vi "SlaveFrame.vi"(0 "buf":u8[](array[numeric]) format="%02x", 5 "数组大小":i32, 7 "Mode":bool) -> (1 "数据帧分析":string, 2 "接收显示":string, 3 "校验成功":bool, 4 "从机编号":u8 format="%02x", 6 "功能码":u8 format="%02x", 8 "起始地址":u16 format="%04x", 10 "寄存器/线圈数量":u16 format="%04x", 14 "数据值索引":u16 format="%04x", 15 "输入数量/字节数":u16 format="%04x")   [LabVIEW 2015]
doc: "Mode = 1? RTU；ASCII;"
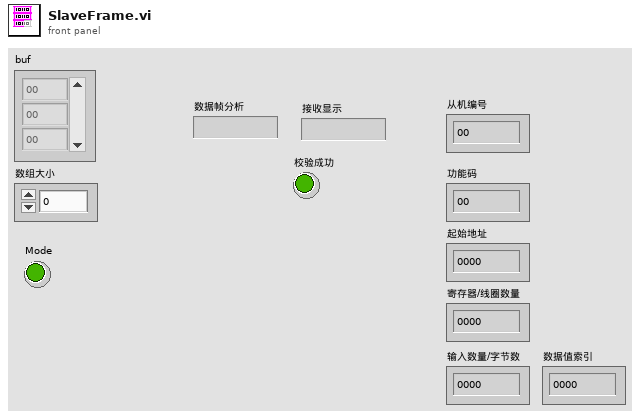
[diagram p1: front panel]
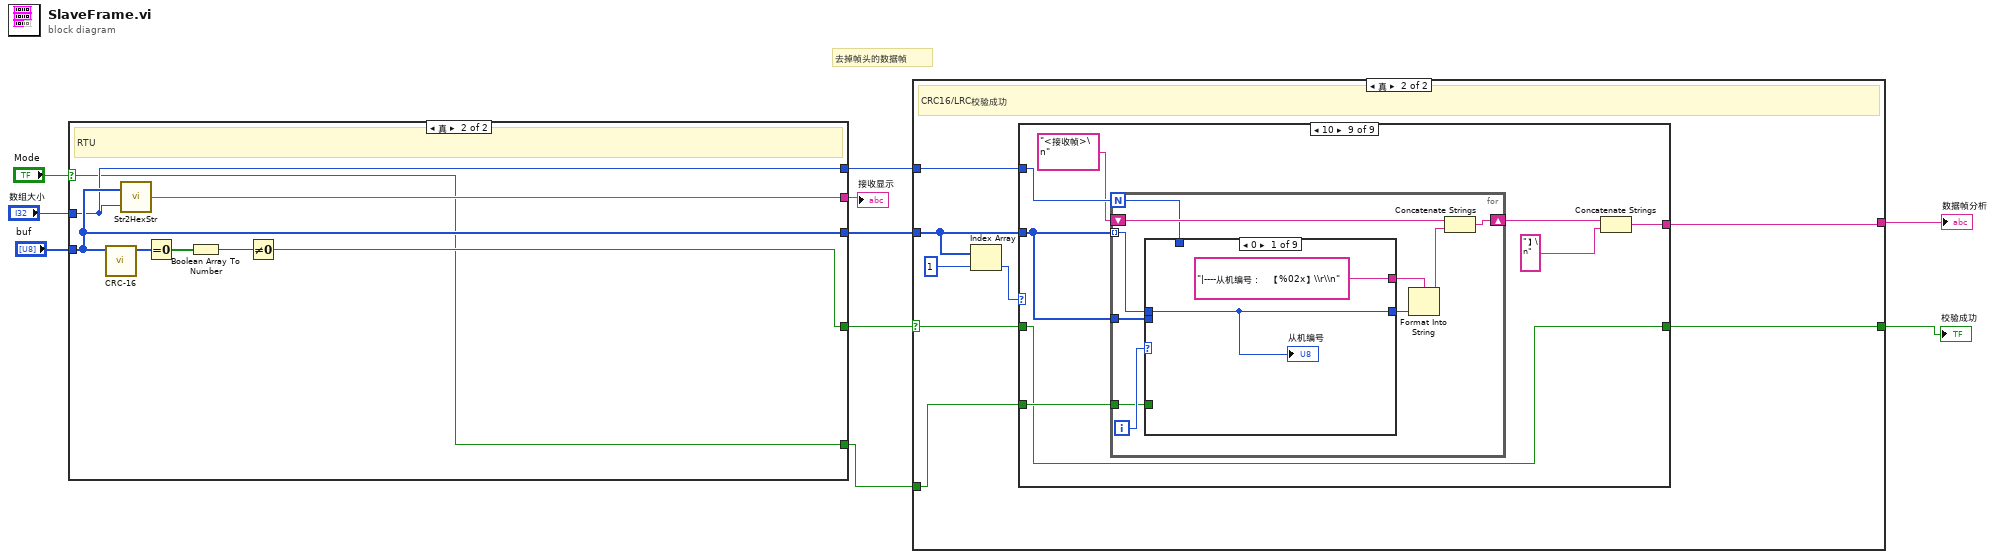
[diagram p0: block diagram]
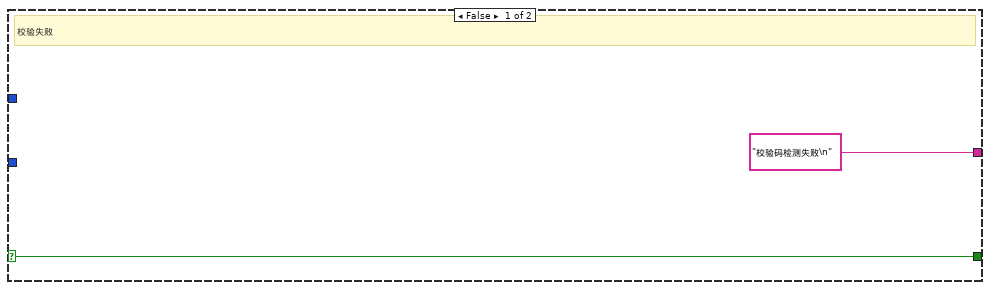
[diagram p2: hidden frame]
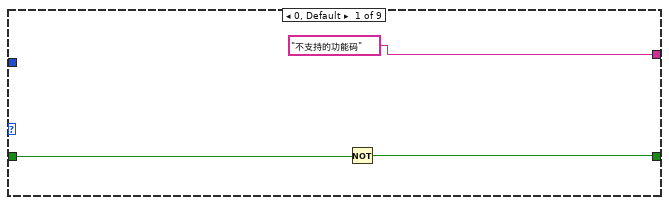
[diagram p3: hidden frame]
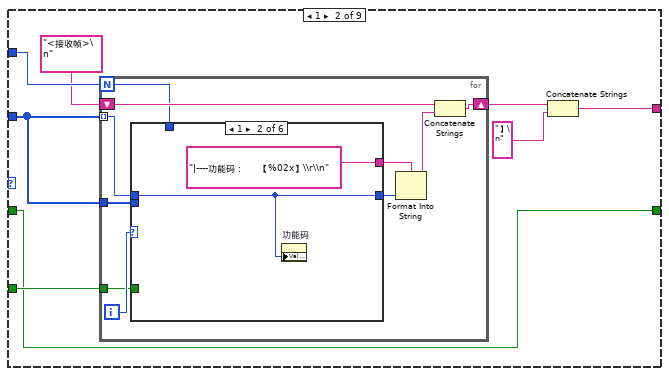
[diagram p4: hidden frame]
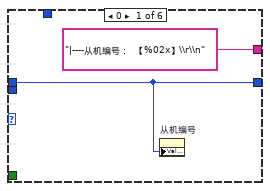
[diagram p5: hidden frame]
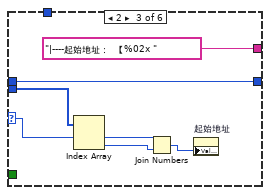
[diagram p6: hidden frame]
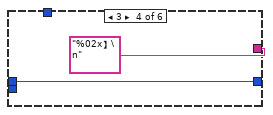
[diagram p7: hidden frame]
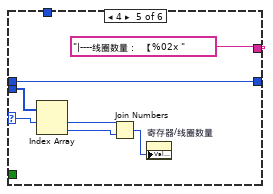
[diagram p8: hidden frame]
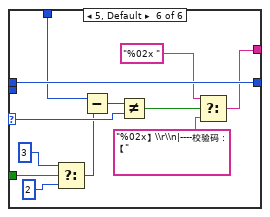
[diagram p9: hidden frame]
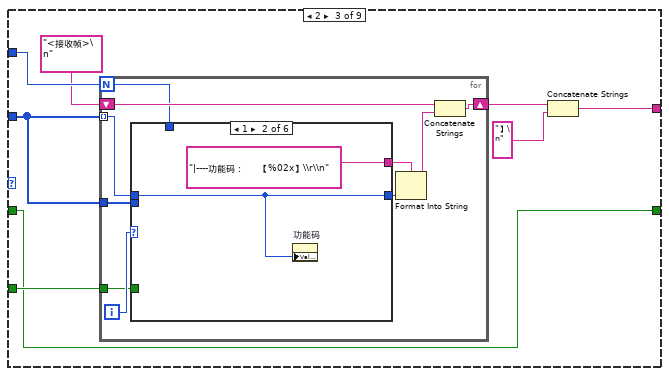
[diagram p10: hidden frame]
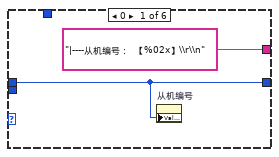
[diagram p11: hidden frame]
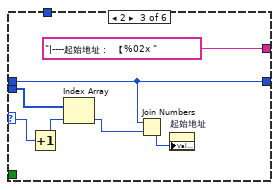
[diagram p12: hidden frame]
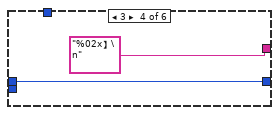
[diagram p13: hidden frame]
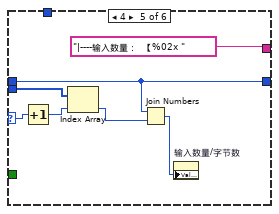
[diagram p14: hidden frame]
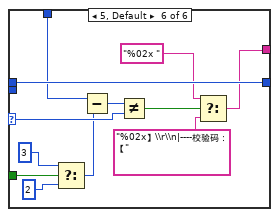
[diagram p15: hidden frame]
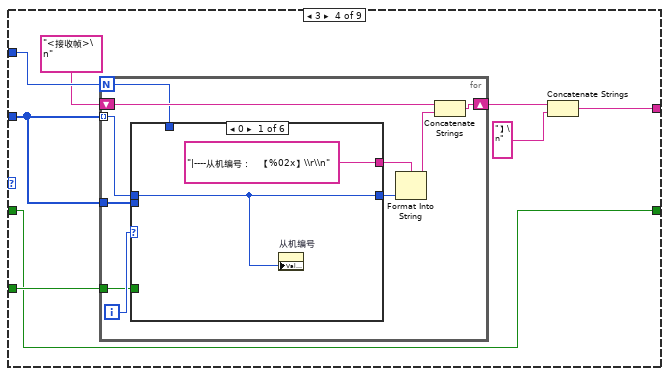
[diagram p16: hidden frame]
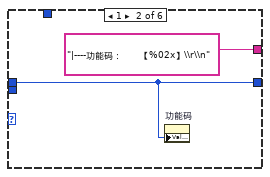
[diagram p17: hidden frame]
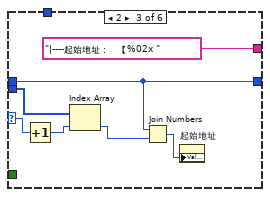
[diagram p18: hidden frame]
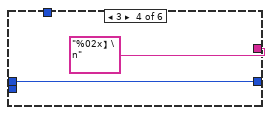
[diagram p19: hidden frame]
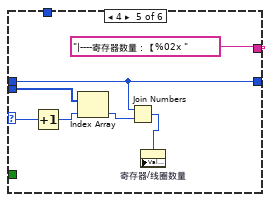
[diagram p20: hidden frame]
diagram:
  # "去掉帧头的数据帧"
  n1 = case shown="真" "Mode" {
    selector: "Mode" -> [w11 w46]
    tunnel: "buf" -> [w24 w48]
    tunnel: "数组大小" -> [_ w47]
    tunnel: [w15 w50] -> w9
    tunnel: [w14 w49] -> w2
    tunnel: [w13 w48] -> w8
    tunnel: [w12 w47] -> w6
    tunnel: [w11 w46] -> w3
    frame False {
      # "ASCII模式"
      n2 = Byte Array To String(unsigned byte array=w24) -> (string=w23:string)
      n3 = Match Pattern(string=w23, regular expression="[:]+[^]+[\\r\\n]") -> (match substring=w15:string)  [unwired: 1 in, 3 out]
      n4 = Match Pattern(string=w23, regular expression="[~:]+[^]+[~\\r\\n]") -> (match substring=w18:string)  [unwired: 1 in, 3 out]
      n5 = String To Byte Array(string=w18) -> (unsigned byte array=w21:u8[])
      n6 = Decimate 1D Array(w21) -> (w20:u8[], w19:u8[])
      n7 = for {
        tunnel: w20 -> [w32] mode=indexing
        tunnel: w19 -> [w30] mode=indexing
        tunnel: [w25] -> w13 mode=indexing
        w29 = u8 57
        w28 = u8 48
        n8 = In Range and Coerce(upper limit=w29, x=w32, lower limit=w28) -> (In Range?=w33:bool)  [unwired: 1 out]
        n9 = In Range and Coerce(upper limit=w29, x=w30, lower limit=w28) -> (In Range?=w31:bool)  [unwired: 1 out]
        n10 = case shown="假" w33 {
          tunnel: w32 -> [w41 w45]
          tunnel: w28 -> [_ w44]
          tunnel: [w40 w43] -> w27
          frame False {
            n11 = Subtract(x=w41, y=u8 55) -> (x-y=w40:u8)
          }
          frame True {
            n12 = Subtract(x=w45, y=w44) -> (x-y=w43:u8)
          }
        }
        n13 = case shown="假" w31 {
          tunnel: w30 -> [w35 w39]
          tunnel: [w34 w38] -> w26
          tunnel: w28 -> [_ w37]
          frame False {
            n14 = Subtract(x=w35, y=u8 55) -> (x-y=w34:u8)
          }
          frame True {
            n15 = Subtract(x=w39, y=w37) -> (x-y=w38:u8)
          }
        }
        n16 = formula code="uInt8 result;\nHi<<=4;\nresult=Hi|Lo;"("Hi"=w27, "Lo"=w26) -> ("result"=w25:u8)
      }
      n17 = Array Size(array=w13) -> (size(s)=w12:i32)
      n18 = call "LRC-8.vi"("Frame in"=w13) -> ("LRC-8"=w16:u8)  [unwired: 2 in]
      n19 = Equal To 0?(x=w16) -> (x = 0?=w14:bool)
    }
    frame True {
      # "RTU"
      n20 = call "CRC-16.vi"("Frame in"=w48) -> ("CRC-16"=w53:u8[])  [unwired: 6 in]
      n21 = call "Str2HexStr.vi"("数组大小"=w47, "数组"=w48) -> ("OutStr"=w50:string)
      n22 = Equal To 0?(x=w53) -> (x = 0?=w52:bool[])
      n23 = Boolean Array To Number(Boolean array=w52) -> (number=w51:u32)
      n24 = Not Equal To 0?(x=w51) -> (x != 0?=w49:bool)
    }
  }
  "接收显示" <- w9
  n25 = case shown="真" w2 {
    selector: w2 -> [w54 w56]
    tunnel: w8 -> [_ w60]
    tunnel: ["校验码检测失败\n" w63] -> w5
    tunnel: w6 -> [_ w62]
    tunnel: w3 -> [_ w61]
    tunnel: [w54 w57] -> w1
    frame False {
      # "校验失败"
    }
    frame True {
      # "CRC16/LRC校验成功"
      n26 = Index Array(array=w60, index=1) -> (element=w58:u8)
      n27 = case shown="10" w58 {
        tunnel: ["不支持的功能码" w74 w124 w174 w224 w274 w320 w366 w430] -> w63
        tunnel: w62 -> [_ w73 w123 w173 w223 w273 w319 w365 w429]
        tunnel: w61 -> [_ w72 w122 w172 w222 w272 w318 w364 w428]
        tunnel: w60 -> [_ w71 w121 w171 w221 w271 w317 w363 w427]
        tunnel: [w64 w67 w117 w167 w217 w267 w313 w359 w423] -> w57
        tunnel: w56 -> [w65 w67 w117 w167 w217 w267 w313 w359 w423]
        frame 0, Default {
          n28 = Not(x=w65) -> (.not. x?=w64:bool)
        }
        frame 1 {
          n29 = for {
            N: w73 -> [w76]
            shift-right: [w84] -> w69
            shift-left: "<接收帧>\n" -> [w83]
            tunnel: w71 -> [w77] mode=indexing
            tunnel: w71 -> [w79]
            tunnel: w72 -> [w75]
            i -> [w80]
            n30 = case shown="1" w80 {
              selector: w80 -> [_ _ w93 _ w100 w109]
              tunnel: ["|----从机编号：  【%02x】\\r\\n" "|----功能码：     【%02x】\\r\\n" "|----起始地址：  【%02x " "%02x】\n" "|----线圈数量：  【%02x " w111] -> w82
              tunnel: w79 -> [_ _ w92 _ w99 _]
              tunnel: [w85 w87 w95 w96 w103 w116] -> w78
              tunnel: w77 -> [w85 w87 w95 w96 w103 w116]
              tunnel: w76 -> [_ _ _ _ _ w115]
              tunnel: w75 -> [_ _ _ _ _ w108]
              frame 0 {
                n31 = property on="从机编号" class="DigNum (严格)"("Value"=w85) -> ()  [unwired: 2 in, 2 out]
              }
              frame 1 {
                n32 = property on="功能码" class="DigNum (严格)"("Value"=w87) -> ()  [unwired: 2 in, 2 out]
              }
              frame 2 {
                n33 = Index Array(array=w92, index #1=w93) -> (element #1=w91:u8, element #2=w90:u8)  [unwired: 1 in]
                n34 = Join Numbers(hi=w91, lo=w90) -> ((hi.lo)=w89:u16)
                n35 = property on="起始地址" class="DigNum (严格)"("Value"=w89) -> ()  [unwired: 2 in, 2 out]
              }
              frame 3 {
              }
              frame 4 {
                n36 = Index Array(array=w99, index #1=w100) -> (element #1=w102:u8, element #2=w101:u8)  [unwired: 1 in]
                n37 = Join Numbers(hi=w102, lo=w101) -> ((hi.lo)=w98:u16)
                n38 = property on="寄存器/线圈数量" class="DigNum (严格)"("Value"=w98) -> ()  [unwired: 2 in, 2 out]
              }
              frame 5, Default {
                n39 = Select(t=3, s=w108, f=2) -> (s? t:f=w106:i32)
                n40 = Subtract(x=w115, y=w106) -> (x-y=w114:i32)
                n41 = Not Equal?(x=w114, y=w109) -> (x != y?=w113:bool)
                n42 = Select(t="%02x ", s=w113, f="%02x】\\r\\n|----校验码：     【") -> (s? t:f=w111:string)
              }
            }
            n43 = Format Into String(format string=w82, w78) -> (resulting string=w81:string)  [unwired: 2 in, 1 out]
            n44 = Concatenate Strings(w83, w81) -> (w84:string)
          }
          n45 = Concatenate Strings(w69, "】\n") -> (w74:string)
        }
        frame 2 {
          n46 = for {
            N: w123 -> [w126]
            shift-right: [w134] -> w119
            shift-left: "<接收帧>\n" -> [w133]
            tunnel: w121 -> [w127] mode=indexing
            tunnel: w121 -> [w129]
            tunnel: w122 -> [w125]
            i -> [w130]
            n47 = case shown="1" w130 {
              selector: w130 -> [_ _ w142 _ w151 w159]
              tunnel: ["|----从机编号：  【%02x】\\r\\n" "|----功能码：     【%02x】\\r\\n" "|----起始地址：  【%02x " "%02x】\n" "|----输入数量：  【%02x " w161] -> w132
              tunnel: w129 -> [_ _ w144 _ w150 _]
              tunnel: [w135 w137 w139 w146 w149 w166] -> w128
              tunnel: w127 -> [w135 w137 w139 w146 w149 w166]
              tunnel: w126 -> [_ _ _ _ _ w165]
              tunnel: w125 -> [_ _ _ _ _ w158]
              frame 0 {
                n48 = property on="从机编号" class="DigNum (严格)"("Value"=w135) -> ()  [unwired: 2 in, 2 out]
              }
              frame 1 {
                n49 = property on="功能码" class="DigNum (严格)"("Value"=w137) -> ()  [unwired: 2 in, 2 out]
              }
              frame 2 {
                n50 = Increment(x=w142) -> (x+1=w141:i32)
                n51 = Index Array(array=w144, index=w141) -> (element=w140:u8)
                n52 = Join Numbers(hi=w139, lo=w140) -> ((hi.lo)=w143:u16)
                n53 = property on="起始地址" class="DigNum (严格)"("Value"=w143) -> ()  [unwired: 2 in, 2 out]
              }
              frame 3 {
              }
              frame 4 {
                n54 = Increment(x=w151) -> (x+1=w153:i32)
                n55 = Index Array(array=w150, index=w153) -> (element=w152:u8)
                n56 = Join Numbers(hi=w149, lo=w152) -> ((hi.lo)=w148:u16)
                n57 = property on="输入数量/字节数" class="DigNum (严格)"("Value"=w148) -> ()  [unwired: 2 in, 2 out]
              }
              frame 5, Default {
                n58 = Select(t=3, s=w158, f=2) -> (s? t:f=w156:i32)
                n59 = Subtract(x=w165, y=w156) -> (x-y=w164:i32)
                n60 = Not Equal?(x=w164, y=w159) -> (x != y?=w163:bool)
                n61 = Select(t="%02x ", s=w163, f="%02x】\\r\\n|----校验码：     【") -> (s? t:f=w161:string)
              }
            }
            n62 = Format Into String(format string=w132, w128) -> (resulting string=w131:string)  [unwired: 2 in, 1 out]
            n63 = Concatenate Strings(w133, w131) -> (w134:string)
          }
          n64 = Concatenate Strings(w119, "】\n") -> (w124:string)
        }
        frame 3 {
          n65 = for {
            N: w173 -> [w176]
            shift-right: [w184] -> w169
            shift-left: "<接收帧>\n" -> [w183]
            tunnel: w171 -> [w177] mode=indexing
            tunnel: w171 -> [w179]
            tunnel: w172 -> [w175]
            i -> [w180]
            n66 = case shown="0" w180 {
              selector: w180 -> [_ _ w192 _ w199 w209]
              tunnel: ["|----从机编号：   【%02x】\\r\\n" "|----功能码：      【%02x】\\r\\n" "|----起始地址：   【%02x " "%02x】\n" "|----寄存器数量：【%02x " w211] -> w182
              tunnel: w179 -> [_ _ w191 _ w200 _]
              tunnel: [w185 w187 w190 w196 w201 w216] -> w178
              tunnel: w177 -> [w185 w187 w190 w196 w201 w216]
              tunnel: w176 -> [_ _ _ _ _ w215]
              tunnel: w175 -> [_ _ _ _ _ w208]
              frame 0 {
                n67 = property on="从机编号" class="DigNum (严格)"("Value"=w185) -> ()  [unwired: 2 in, 2 out]
              }
              frame 1 {
                n68 = property on="功能码" class="DigNum (严格)"("Value"=w187) -> ()  [unwired: 2 in, 2 out]
              }
              frame 2 {
                n69 = Increment(x=w192) -> (x+1=w194:i32)
                n70 = Index Array(array=w191, index=w194) -> (element=w193:u8)
                n71 = Join Numbers(hi=w190, lo=w193) -> ((hi.lo)=w189:u16)
                n72 = property on="起始地址" class="DigNum (严格)"("Value"=w189) -> ()  [unwired: 2 in, 2 out]
              }
              frame 3 {
              }
              frame 4 {
                n73 = Increment(x=w199) -> (x+1=w203:i32)
                n74 = Index Array(array=w200, index=w203) -> (element=w202:u8)
                n75 = Join Numbers(hi=w201, lo=w202) -> ((hi.lo)=w198:u16)
                n76 = property on="寄存器/线圈数量" class="DigNum (严格)"("Value"=w198) -> ()  [unwired: 2 in, 2 out]
              }
              frame 5, Default {
                n77 = Select(t=3, s=w208, f=2) -> (s? t:f=w206:i32)
                n78 = Subtract(x=w215, y=w206) -> (x-y=w214:i32)
                n79 = Not Equal?(x=w214, y=w209) -> (x != y?=w213:bool)
                n80 = Select(t="%02x ", s=w213, f="%02x】\\r\\n|----校验码：      【") -> (s? t:f=w211:string)
              }
            }
            n81 = Format Into String(format string=w182, w178) -> (resulting string=w181:string)  [unwired: 2 in, 1 out]
            n82 = Concatenate Strings(w183, w181) -> (w184:string)
          }
          n83 = Concatenate Strings(w169, "】\n") -> (w174:string)
        }
        frame 4 {
          n84 = for {
            N: w223 -> [w226]
            shift-right: [w234] -> w219
            shift-left: "<接收帧>\n" -> [w233]
            tunnel: w221 -> [w227] mode=indexing
            tunnel: w221 -> [w229]
            tunnel: w222 -> [w225]
            i -> [w230]
            n85 = case shown="5, 默认" w230 {
              selector: w230 -> [_ _ w241 _ w248 w259]
              tunnel: ["|----从机编号：   【%02x】\\r\\n" "|----功能码：      【%02x】\\r\\n" "|----起始地址：   【%02x " "%02x】\n" "|----寄存器数量：【%02x " w261] -> w232
              tunnel: w229 -> [_ _ w240 _ w249 _]
              tunnel: [w235 w237 w239 w246 w250 w266] -> w228
              tunnel: w227 -> [w235 w237 w239 w246 w250 w266]
              tunnel: w226 -> [_ _ _ _ _ w265]
              tunnel: w225 -> [_ _ _ _ _ w258]
              frame 0 {
                n86 = property on="从机编号" class="DigNum (严格)"("Value"=w235) -> ()  [unwired: 2 in, 2 out]
              }
              frame 1 {
                n87 = property on="功能码" class="DigNum (严格)"("Value"=w237) -> ()  [unwired: 2 in, 2 out]
              }
              frame 2 {
                n88 = Increment(x=w241) -> (x+1=w243:i32)
                n89 = Index Array(array=w240, index=w243) -> (element=w242:u8)
                n90 = Join Numbers(hi=w239, lo=w242) -> ((hi.lo)=w244:u16)
                n91 = property on="起始地址" class="DigNum (严格)"("Value"=w244) -> ()  [unwired: 2 in, 2 out]
              }
              frame 3 {
              }
              frame 4 {
                n92 = Increment(x=w248) -> (x+1=w253:i32)
                n93 = Index Array(array=w249, index=w253) -> (element=w252:u8)
                n94 = Join Numbers(hi=w250, lo=w252) -> ((hi.lo)=w251:u16)
                n95 = property on="寄存器/线圈数量" class="DigNum (严格)"("Value"=w251) -> ()  [unwired: 2 in, 2 out]
              }
              frame 5, Default {
                n96 = Select(t=3, s=w258, f=2) -> (s? t:f=w256:i32)
                n97 = Subtract(x=w265, y=w256) -> (x-y=w264:i32)
                n98 = Not Equal?(x=w264, y=w259) -> (x != y?=w263:bool)
                n99 = Select(t="%02x ", s=w263, f="%02x】\\r\\n|----校验码：      【") -> (s? t:f=w261:string)
              }
            }
            n100 = Format Into String(format string=w232, w228) -> (resulting string=w231:string)  [unwired: 2 in, 1 out]
            n101 = Concatenate Strings(w233, w231) -> (w234:string)
          }
          n102 = Concatenate Strings(w219, "】\n") -> (w224:string)
        }
        frame 5 {
          n103 = for {
            N: w273 -> [w276]
            shift-right: [w284] -> w269
            shift-left: "<接收帧>\n" -> [w283]
            tunnel: w271 -> [w277] mode=indexing
            tunnel: w271 -> [w279]
            tunnel: w272 -> [w275]
            i -> [w280]
            n104 = case shown="0" w280 {
              selector: w280 -> [_ _ w291 _ w298 w305]
              tunnel: ["|----从机编号：   【%02x】\\r\\n" "|----功能码：      【%02x】\\r\\n" "|----起始地址：   【%02x " "%02x】\n" "|----数据值：      【%02x " w307] -> w282
              tunnel: w279 -> [_ _ w290 _ _ _]
              tunnel: [w285 w287 w289 w296 w299 w312] -> w278
              tunnel: w277 -> [w285 w287 w289 w296 w299 w312]
              tunnel: w276 -> [_ _ _ _ _ w311]
              tunnel: w275 -> [_ _ _ _ _ w304]
              frame 0 {
                n105 = property on="从机编号" class="DigNum (严格)"("Value"=w285) -> ()  [unwired: 2 in, 2 out]
              }
              frame 1 {
                n106 = property on="功能码" class="DigNum (严格)"("Value"=w287) -> ()  [unwired: 2 in, 2 out]
              }
              frame 2 {
                n107 = Increment(x=w291) -> (x+1=w293:i32)
                n108 = Index Array(array=w290, index=w293) -> (element=w292:u8)
                n109 = Join Numbers(hi=w289, lo=w292) -> ((hi.lo)=w294:u16)
                n110 = property on="起始地址" class="DigNum (严格)"("Value"=w294) -> ()  [unwired: 2 in, 2 out]
              }
              frame 3 {
              }
              frame 4 {
                n111 = property on="数据值索引" class="DigNum (严格)"("Value"=w298) -> ()  [unwired: 2 in, 2 out]
              }
              frame 5, Default {
                n112 = Select(t=3, s=w304, f=2) -> (s? t:f=w302:i32)
                n113 = Subtract(x=w311, y=w302) -> (x-y=w310:i32)
                n114 = Not Equal?(x=w310, y=w305) -> (x != y?=w309:bool)
                n115 = Select(t="%02x ", s=w309, f="%02x】\\r\\n|----校验码：      【") -> (s? t:f=w307:string)
              }
            }
            n116 = Format Into String(format string=w282, w278) -> (resulting string=w281:string)  [unwired: 2 in, 1 out]
            n117 = Concatenate Strings(w283, w281) -> (w284:string)
          }
          n118 = Concatenate Strings(w269, "】\n") -> (w274:string)
        }
        frame 6 {
          n119 = for {
            N: w319 -> [w322]
            shift-right: [w330] -> w315
            shift-left: "<接收帧>\n" -> [w329]
            tunnel: w317 -> [w323] mode=indexing
            tunnel: w317 -> [w325]
            tunnel: w318 -> [w321]
            i -> [w326]
            n120 = case shown="0" w326 {
              selector: w326 -> [_ _ w337 _ w344 w351]
              tunnel: ["|----从机编号：   【%02x】\\r\\n" "|----功能码：      【%02x】\\r\\n" "|----寄存器地址：【%02x " "%02x】\n" "|----寄存器值：   【%02x " w353] -> w328
              tunnel: w325 -> [_ _ w336 _ _ _]
              tunnel: [w331 w333 w335 w342 w345 w358] -> w324
              tunnel: w323 -> [w331 w333 w335 w342 w345 w358]
              tunnel: w322 -> [_ _ _ _ _ w357]
              tunnel: w321 -> [_ _ _ _ _ w350]
              frame 0 {
                n121 = property on="从机编号" class="DigNum (严格)"("Value"=w331) -> ()  [unwired: 2 in, 2 out]
              }
              frame 1 {
                n122 = property on="功能码" class="DigNum (严格)"("Value"=w333) -> ()  [unwired: 2 in, 2 out]
              }
              frame 2 {
                n123 = Increment(x=w337) -> (x+1=w339:i32)
                n124 = Index Array(array=w336, index=w339) -> (element=w338:u8)
                n125 = Join Numbers(hi=w335, lo=w338) -> ((hi.lo)=w340:u16)
                n126 = property on="起始地址" class="DigNum (严格)"("Value"=w340) -> ()  [unwired: 2 in, 2 out]
              }
              frame 3 {
              }
              frame 4 {
                n127 = property on="数据值索引" class="DigNum (严格)"("Value"=w344) -> ()  [unwired: 2 in, 2 out]
              }
              frame 5, Default {
                n128 = Select(t=3, s=w350, f=2) -> (s? t:f=w348:i32)
                n129 = Subtract(x=w357, y=w348) -> (x-y=w356:i32)
                n130 = Not Equal?(x=w356, y=w351) -> (x != y?=w355:bool)
                n131 = Select(t="%02x ", s=w355, f="%02x】\\r\\n|----校验码：      【") -> (s? t:f=w353:string)
              }
            }
            n132 = Format Into String(format string=w328, w324) -> (resulting string=w327:string)  [unwired: 2 in, 1 out]
            n133 = Concatenate Strings(w329, w327) -> (w330:string)
          }
          n134 = Concatenate Strings(w315, "】\n") -> (w320:string)
        }
        frame 15 {
          n135 = for {
            N: w365 -> [w368]
            shift-right: [w376] -> w361
            shift-left: "<接收帧>\n" -> [w375]
            tunnel: w363 -> [w369] mode=indexing
            tunnel: w363 -> [w371]
            tunnel: w364 -> [w367]
            i -> [w372]
            n136 = case shown="8, 默认" w372 {
              selector: w372 -> [_ _ w383 _ w393 _ _ w401 w415]
              tunnel: ["|----从机编号：   【%02x】\\r\\n" "|----功能码：      【%02x】\\r\\n" "|----起始地址：   【%02x " "%02x】\n" "|----输出数量：   【%02x " "%02x】\n" "|----字节数：      【%02x】 \\r\\n" w403 w417] -> w374
              tunnel: w371 -> [_ _ w382 _ w392 _ _ w408 _]
              tunnel: [w377 w379 w381 w388 w391 w397 w399 w410 w422] -> w370
              tunnel: w369 -> [w377 w379 w381 w388 w391 w397 w399 w410 w422]
              tunnel: w368 -> [_ _ _ _ _ _ _ _ w421]
              tunnel: w367 -> [_ _ _ _ _ _ _ _ w414]
              frame 0 {
                n137 = property on="从机编号" class="DigNum (严格)"("Value"=w377) -> ()  [unwired: 2 in, 2 out]
              }
              frame 1 {
                n138 = property on="功能码" class="DigNum (严格)"("Value"=w379) -> ()  [unwired: 2 in, 2 out]
              }
              frame 2 {
                n139 = Increment(x=w383) -> (x+1=w385:i32)
                n140 = Index Array(array=w382, index=w385) -> (element=w384:u8)
                n141 = Join Numbers(hi=w381, lo=w384) -> ((hi.lo)=w386:u16)
                n142 = property on="起始地址" class="DigNum (严格)"("Value"=w386) -> ()  [unwired: 2 in, 2 out]
              }
              frame 3 {
              }
              frame 4 {
                n143 = Increment(x=w393) -> (x+1=w395:i32)
                n144 = Index Array(array=w392, index=w395) -> (element=w394:u8)
                n145 = Join Numbers(hi=w391, lo=w394) -> ((hi.lo)=w390:u16)
                n146 = property on="寄存器/线圈数量" class="DigNum (严格)"("Value"=w390) -> ()  [unwired: 2 in, 2 out]
              }
              frame 5 {
              }
              frame 6 {
                n147 = property on="输入数量/字节数" class="DigNum (严格)"("Value"=w399) -> ()  [unwired: 2 in, 2 out]
              }
              frame 7 {
                n148 = Decrement(x=w401) -> (x-1=w409:i32)
                n149 = Index Array(array=w408, index=w409) -> (element=w407:u8)
                n150 = Greater?(x=w407, y=1) -> (0:w405:bool)
                n151 = Select(t="|----数据值：      【%02x ", s=w405, f="|----数据值：      【%02x】\n|----校验码：      【") -> (s? t:f=w403:string)
                n152 = property on="数据值索引" class="DigNum (严格)"("Value"=w401) -> ()  [unwired: 2 in, 2 out]
              }
              frame 8, Default {
                n153 = Select(t=3, s=w414, f=2) -> (s? t:f=w412:i32)
                n154 = Subtract(x=w421, y=w412) -> (x-y=w420:i32)
                n155 = Not Equal?(x=w420, y=w415) -> (x != y?=w419:bool)
                n156 = Select(t="%02x ", s=w419, f="%02x】\\r\\n|----校验码：      【") -> (s? t:f=w417:string)
              }
            }
            n157 = Format Into String(format string=w374, w370) -> (resulting string=w373:string)  [unwired: 2 in, 1 out]
            n158 = Concatenate Strings(w375, w373) -> (w376:string)
          }
          n159 = Concatenate Strings(w361, "】\n") -> (w366:string)
        }
        frame 16 {
          n160 = for {
            N: w429 -> [w432]
            shift-right: [w440] -> w425
            shift-left: "<接收帧>\n" -> [w439]
            tunnel: w427 -> [w433] mode=indexing
            tunnel: w427 -> [w435]
            tunnel: w428 -> [w431]
            i -> [w436]
            n161 = case shown="0" w436 {
              selector: w436 -> [_ _ w448 _ w457 _ _ w465 w472]
              tunnel: ["|----从机编号：   【%02x】\\r\\n" "|----功能码：      【%02x】\\r\\n" "|----起始地址：   【%02x " "%02x】\n" "|----寄存器数量：【%02x " "%02x】\n" "|----字节数：      【%02x】 \\r\\n" "|----数据值：      【%02x " w474] -> w438
              tunnel: w435 -> [_ _ w450 _ w456 _ _ _ _]
              tunnel: [w441 w443 w445 w452 w455 w461 w463 w467 w479] -> w434
              tunnel: w433 -> [w441 w443 w445 w452 w455 w461 w463 w467 w479]
              tunnel: w432 -> [_ _ _ _ _ _ _ _ w478]
              tunnel: w431 -> [_ _ _ _ _ _ _ _ w471]
              frame 0 {
                "从机编号" <- w441
              }
              frame 1 {
                "功能码" <- w443
              }
              frame 2 {
                n162 = Increment(x=w448) -> (x+1=w447:i32)
                n163 = Index Array(array=w450, index=w447) -> (element=w446:u8)
                n164 = Join Numbers(hi=w445, lo=w446) -> ((hi.lo)=→"起始地址":u16)
              }
              frame 3 {
              }
              frame 4 {
                n165 = Increment(x=w457) -> (x+1=w459:i32)
                n166 = Index Array(array=w456, index=w459) -> (element=w458:u8)
                n167 = Join Numbers(hi=w455, lo=w458) -> ((hi.lo)=→"寄存器/线圈数量":u16)
              }
              frame 5 {
              }
              frame 6 {
                "输入数量/字节数" <- w463
              }
              frame 7 {
                "数据值索引" <- w465
              }
              frame 8, Default {
                n168 = Select(t=3, s=w471, f=2) -> (s? t:f=w469:i32)
                n169 = Subtract(x=w478, y=w469) -> (x-y=w477:i32)
                n170 = Not Equal?(x=w477, y=w472) -> (x != y?=w476:bool)
                n171 = Select(t="%02x ", s=w476, f="%02x】\\r\\n|----校验码：      【") -> (s? t:f=w474:string)
              }
            }
            n172 = Format Into String(format string=w438, w434) -> (resulting string=w437:string)  [unwired: 2 in, 1 out]
            n173 = Concatenate Strings(w439, w437) -> (w440:string)
          }
          n174 = Concatenate Strings(w425, "】\n") -> (w430:string)
        }
      }
    }
  }
  "数据帧分析" <- w5
  "校验成功" <- w1
